vi "Set Switch.vi"(8 "error in (no error)":errorcluster, 10 "Switch Settings":bool[](array[boolean]), 11 "I2C Switch in":refnum<class "I2C Switch.lvclass">) -> (0 "error out":errorcluster, 3 "I2C Switch out":refnum<class "I2C Switch.lvclass">)   [LabVIEW 2020, in "CTI-Peripheral.lvlib" / "I2C Switch.lvclass"]
uses:
  I2C Switch.lvclass
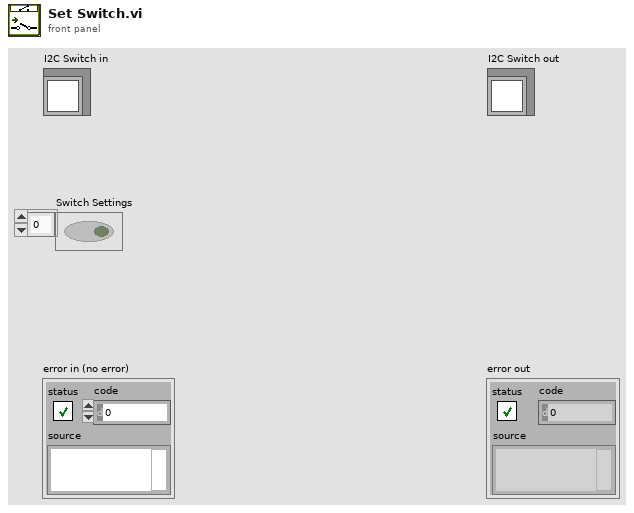
[diagram p1: front panel]
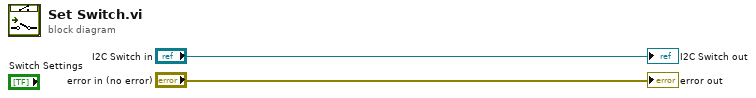
[diagram p0: block diagram]
diagram:
  "error out" <- "error in (no error)"
  "I2C Switch out" <- "I2C Switch in"
